vi "Deadzone.vi"(2 "Deadzone":dbl, 3 "Value":dbl) -> (0 "In Deadzone?":bool, 1 "Value or 0":dbl)   [LabVIEW 2016]
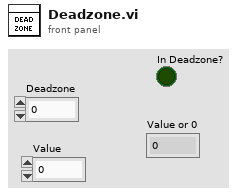
[diagram p1: front panel]
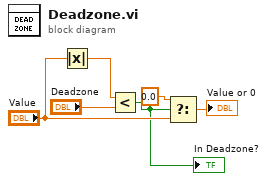
[diagram p0: block diagram]
diagram:
  n1 = Absolute Value(x="Value") -> (abs(x)=w5:dbl)
  n2 = Less?(x=w5, y="Deadzone") -> (x < y?=w1:bool)
  "In Deadzone?" <- w1
  n3 = Select(t=0.0, s=w1, f="Value") -> (s? t:f=→"Value or 0":dbl)
